vi "Clear Directory.vi"(8 "error in":errorcluster) -> (0 "error out":errorcluster)   [LabVIEW 2017, in "TestTextFileSink.lvclass"]
uses:
  TestTextFileSink.lvclass
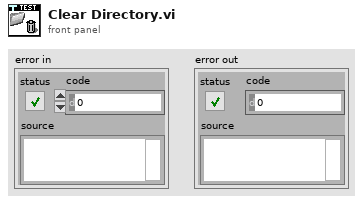
[diagram p1: front panel]
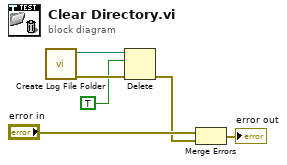
[diagram p0: block diagram]
diagram:
  n1 = call "Create Log File Folder.vi"() -> ("error out"=w5:errorcluster, "Folder Path"=w6:path)  [unwired: 10 in]
  n2 = Delete(path (use dialog)=w6, entire hierarchy (F)=TRUE, error in=w5) -> (error out=w2:errorcluster)  [unwired: 2 in, 2 out]
  n3 = Merge Errors("error in", w2) -> (→"error out":errorcluster)
